vi "采配水全局变量.vi"() -> ()   [LabVIEW 2016, in "PLC.lvlib"]
uses:
  PLC.lvlib
panel:
  out "自动运行状态":string
  in  "报警簇":T1
  out "参数设置":T2
  in  "状态":T3
  out "转换值":T4
  out "AD":T5
  in  "输出状态":T6
  in  "输入状态":T7
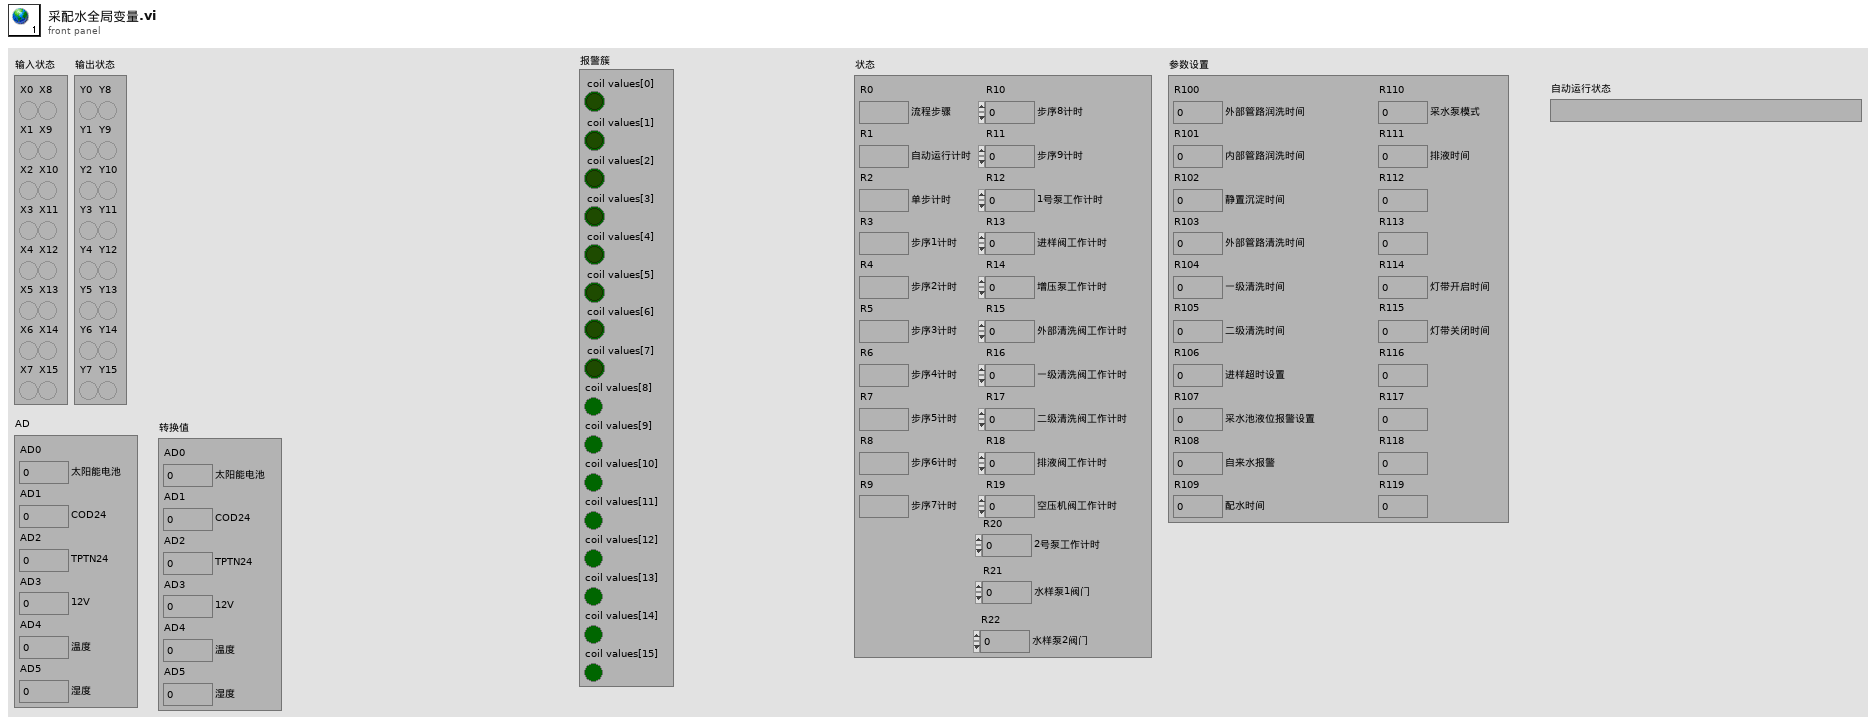
[diagram p1: front panel]
types:
  T1 = cluster{"coil values[0]":bool, "coil values[1]":bool, "coil values[2]":bool, "coil values[3]":bool, "coil values[4]":bool, "coil values[5]":bool, "coil values[6]":bool, "coil values[7]":bool, "coil values[8]":bool, "coil values[9]":bool, "coil values[10]":bool, "coil values[11]":bool, "coil values[12]":bool, "coil values[13]":bool, "coil values[14]":bool, "coil values[15]":bool}
  T2 = cluster{"R100":i16, "R101":i16, "R102":i16, "R103":i16, "R104":i16, "R105":i16, "R106":i16, "R107":i16, "R108":i16, "R109":i16, "R110":i16, "R111":i16, "R112":i16, "R113":i16, "R114":i16, "R115":i16, "R116":i16, "R117":i16, "R118":i16, "R119":i16}
  T3 = cluster{"R0":i16, "R1":i16, "R2":i16, "R3":i16, "R4":i16, "R5":i16, "R6":i16, "R7":i16, "R8":i16, "R9":i16, "R10":i16, "R11":i16, "R12":i16, "R13":i16, "R14":i16, "R15":i16, "R16":i16, "R17":i16, "R18":i16, "R19":i16, "R20":i16, "R21":i16, "R22":i16}
  T4 = cluster{"AD0":sgl, "AD1":sgl, "AD2":sgl, "AD3":sgl, "AD4":sgl, "AD5":sgl}
  T5 = cluster{"AD0":i16, "AD1":i16, "AD2":i16, "AD3":i16, "AD4":i16, "AD5":i16}
  T6 = cluster{"Y0":bool, "Y1":bool, "Y2":bool, "Y3":bool, "Y4":bool, "Y5":bool, "Y6":bool, "Y7":bool, "Y8":bool, "Y9":bool, "Y10":bool, "Y11":bool, "Y12":bool, "Y13":bool, "Y14":bool, "Y15":bool}
  T7 = cluster{"X0":bool, "X1":bool, "X2":bool, "X3":bool, "X4":bool, "X5":bool, "X6":bool, "X7":bool, "X8":bool, "X9":bool, "X10":bool, "X11":bool, "X12":bool, "X13":bool, "X14":bool, "X15":bool}
diagram:
